vi "Save Last Folder.vi"(8 "error in (no error)":errorcluster, 10 ".proto Path":path, 11 "Pref Group":refnum<class "Pref Group.lvclass">) -> (0 "error out":errorcluster)   [LabVIEW 2020, in "LV-Protoc.lvlib" / "LV-Protoc.lvclass"]
uses:
  LV-Protoc.lvclass
  lv-userprefs/User Prefs/Pref Group/Pref Group.lvclass
  LV-Protoc.lvclass/LV-Protoc.ctl
  lv-userprefs/User Prefs/PrefsDB/PrefsDB.lvclass
  lv-cdm/CDM-Config/CDM-Config.lvlib
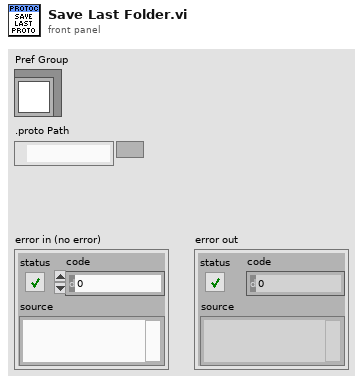
[diagram p1: front panel]
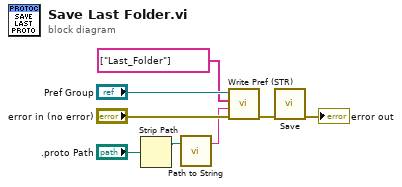
[diagram p0: block diagram]
diagram:
  n1 = Strip Path(path=".proto Path") -> (stripped path=w2:path)  [unwired: 1 out]
  n2 = call "Path to String.vi"("Path"=w2) -> ("Path String"=w1:string)  [unwired: 2 in]
  n3 = call "Write Pref (STR).vi"("error in (no error)"="error in (no error)", "Value"=w1, "Pref Hierarchy"=string[] ["Last_Folder"], "Pref Group in"="Pref Group") -> ("error out"=w4:errorcluster)  [unwired: 6 in, 1 out]
  n4 = call "Save.vi"("error in (no error)"=w4) -> ("error out"=→"error out":errorcluster)  [unwired: 9 in, 1 out]
